vi "_API_TESTER.vi"() -> ()   [LabVIEW 2019, in "_ConfigClass_INI.lvlib" / "_ConfigClass_INI.lvclass"]
uses:
  _ConfigClass_INI.lvclass
panel:
  out "error out":errorcluster
  in  "param_value_in":string
  in  "get":bool
  in  "set":bool
  out "param_value_out":string
  in  "param_in":string
  in  "stop":bool
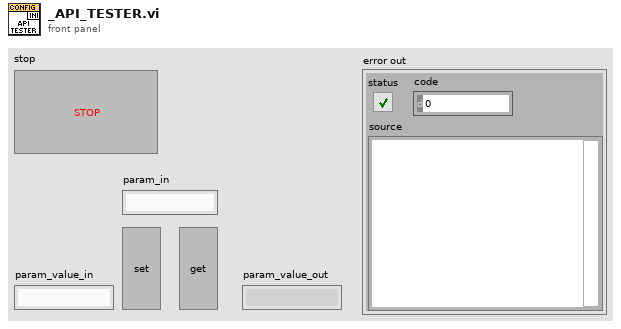
[diagram p1: front panel]
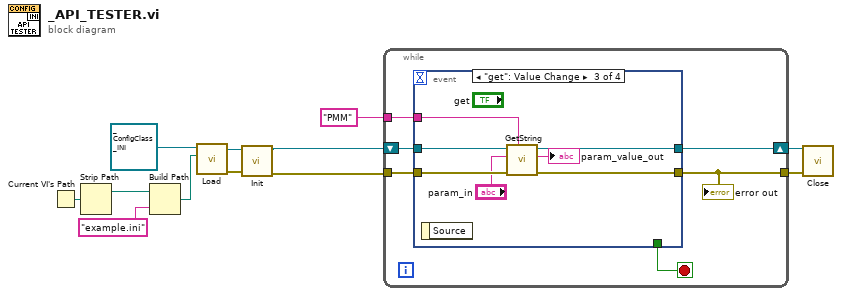
[diagram p0: block diagram]
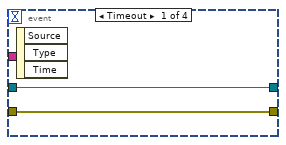
[diagram p2: hidden frame]
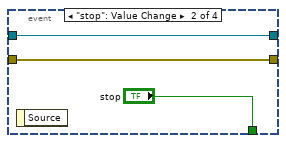
[diagram p3: hidden frame]
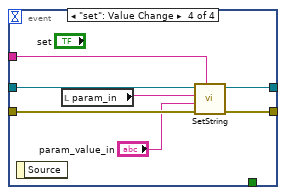
[diagram p4: hidden frame]
diagram:
  n1 = Current VI's Path() -> (path=w7:path)
  n2 = Strip Path(path=w7) -> (stripped path=w6:path)  [unwired: 1 out]
  n3 = Build Path(base path=w6, name or relative path="example.ini") -> (appended path=w4:path)
  n4 = call-dynamic "Load.vi"("Data_IN"=w4, "_ConfigClass_INI_IN"=refnum<class "_ConfigClass_INI.lvclass"> refnum ("_ConfigClass_INI.lvlib:_ConfigClass_INI.lvclass")) -> ("error out"=w10:errorcluster, "_ConfigClass_INI_OUT"=w12:refnum<class "_ConfigClass_INI.lvclass">)  [unwired: 8 in]
  n5 = call-dynamic "Init.vi"("error in (no error)"=w10, "Config.lvlib:_ConfigClass_ApplSett_IN"=w12) -> ("error out"=w2:errorcluster, "Config.lvlib:_ConfigClass_ApplSett_OUT"=w3:refnum<class "_ConfigClass_INI.lvclass">)  [unwired: 8 in]
  n6 = while {
    tunnel: w2 -> [w15]
    tunnel: [w14] -> w8
    shift-right: [w16] -> w9
    shift-left: w3 -> [w17]
    tunnel: "PMM" ("group") -> [w13]
    stop <- w18 stop-if-true
    n7 = event shown="[2] \"get\": Value Change" {
      selector: _ -> [_ _ _ _]
      dyn-events: _ -> [_ _ _ _]
      timeout: _ -> [_ _ _ _]
      tunnel: [_ "stop" _ _] -> w18
      tunnel: w17 -> [w20 w22 w30 w37]
      tunnel: [w20 w22 w29 w36] -> w16
      tunnel: w15 -> [w19 w21 w28 w34]
      tunnel: [w19 w21 w27 w35] -> w14
      tunnel: w13 -> [_ _ w24 w31]
      event Timeout {
        n8 = event-data() -> ()  [unwired: 1 in, 3 out]
      }
      event "stop": Value Change {
        n9 = event-data() -> ()  [unwired: 1 in, 1 out]
      }
      event "get": Value Change {
        n10 = event-data() -> ()  [unwired: 1 in, 1 out]
        n11 = call-dynamic "GetString.vi"("group"=w24, "error in (no error)"=w28, "param"="param_in", "_ConfigClass_INI_IN"=w30) -> ("error out"=w27:errorcluster, "string_out"=→"param_value_out":string, "_ConfigClass_INI_OUT"=w29:refnum<class "_ConfigClass_INI.lvclass">)  [unwired: 5 in]
      }
      event "set": Value Change {
        n12 = event-data() -> ()  [unwired: 1 in, 1 out]
        n13 = local read "param_in"() -> (w32:string)
        n14 = call-dynamic "SetString.vi"("group"=w31, "error in (no error)"=w34, "string_in"="param_value_in", "param"=w32, "_ConfigClass_INI_IN"=w37) -> ("error out"=w35:errorcluster, "_ConfigClass_INI_OUT"=w36:refnum<class "_ConfigClass_INI.lvclass">)  [unwired: 5 in]
      }
    }
    "error out" <- w14
  }
  n15 = call-dynamic "Close.vi"("error in (no error)"=w8, "_ConfigClass_INI_IN"=w9) -> ()  [unwired: 8 in, 2 out]
